vi "PreUUT Dialog.vi"(8 "error in (no error)":errorcluster, 11 "Valid Part Numbers":string[](array[string])) -> (0 "error out":errorcluster, 1 "Comments Out":string, 2 "Part Number Out":string(combo), 3 "Cancelled?":bool, 5 "Serial Number Out":string)   [LabVIEW 2020, in "Common Dialogs.lvlib"]
doc: "Use this template to create a dialog box with event handling."
uses:
  <vilib>/regexp/Match Regular Expression.xnode
  Common Dialogs.lvlib
panel:
  in  "Part Number OK":bool
  in  "Serial Number OK":bool
  in  "Comments":string
  in  "Part Number":string(combo)
  in  "Serial Number":string
  in  "Cancel":bool
  in  "OK":bool
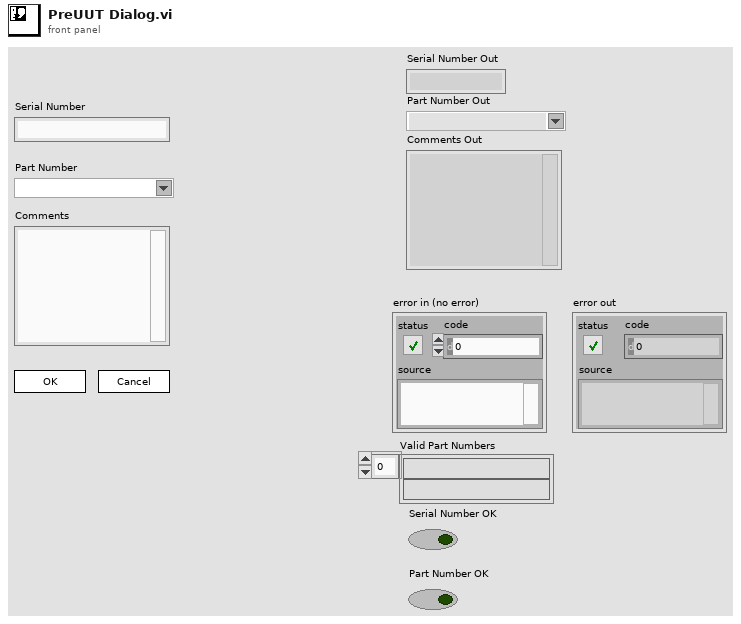
[diagram p1: front panel]
types:
  T1 = enum8{"Enabled", "Disabled", "Disabled and Grayed Out"}
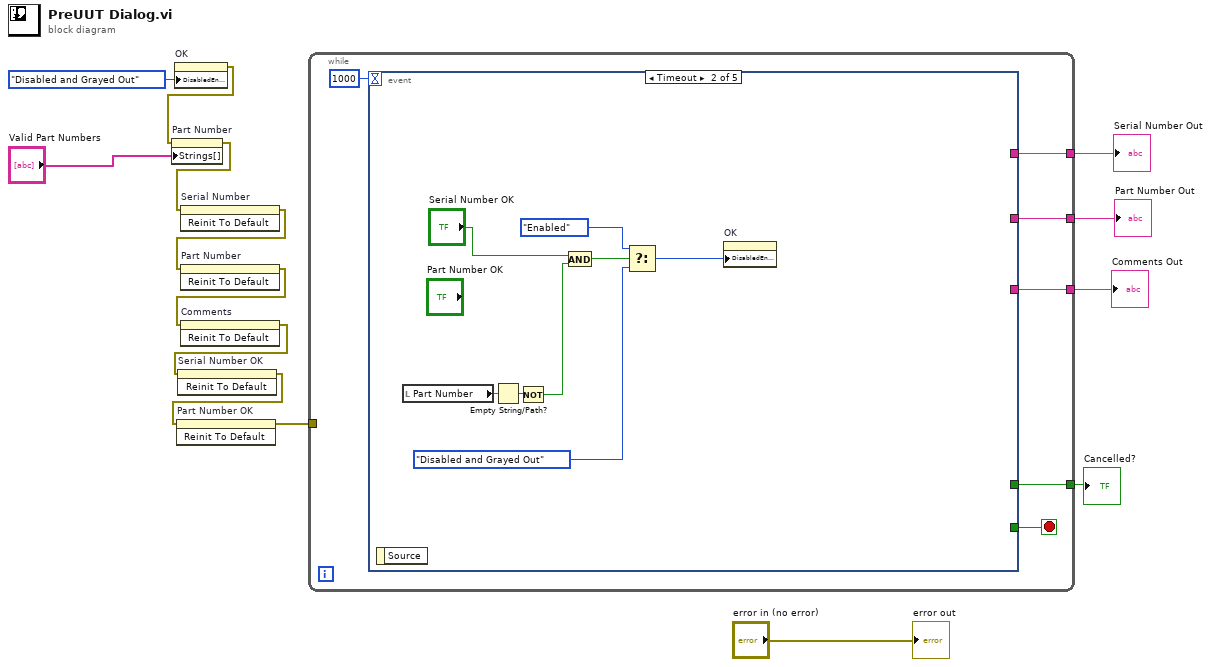
[diagram p0: block diagram]
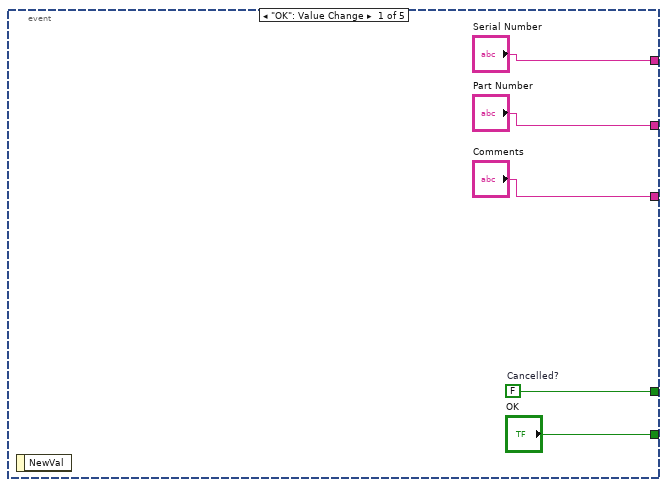
[diagram p2: hidden frame]
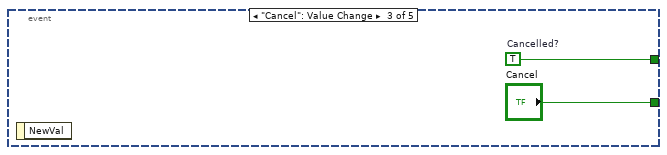
[diagram p3: hidden frame]
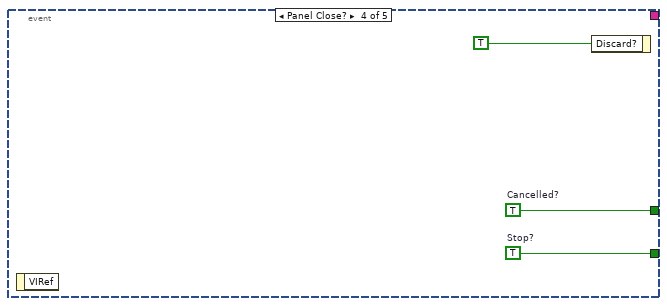
[diagram p4: hidden frame]
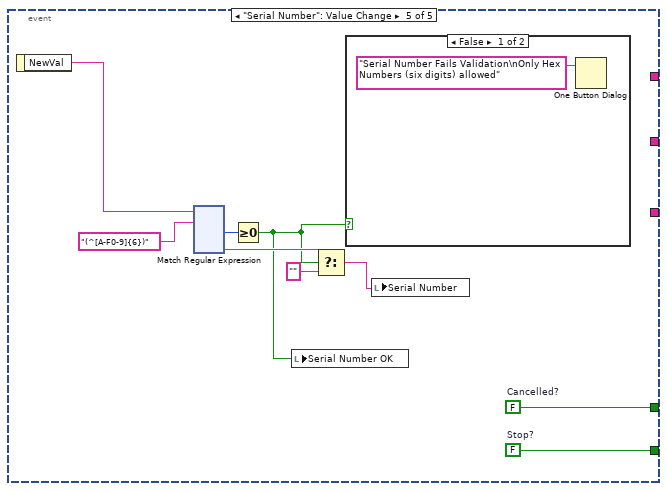
[diagram p5: hidden frame]
diagram:
  n1 = property on="OK" class="Bool"("DisabledEnum"=T1."Disabled and Grayed Out" ("Disabled")) -> (error out=w5:errorcluster)  [unwired: 2 in, 1 out]
  n2 = property on="Part Number" class="CmbBox"(error in=w5, "Strings[]"="Valid Part Numbers") -> (error out=w7:errorcluster)  [unwired: 1 in, 1 out]
  n3 = invoke on="Serial Number" class="Str" method="Reinit To Default"(error in=w7) -> (error out=w9:errorcluster)  [unwired: 2 in, 2 out]
  n4 = invoke on="Part Number" class="CmbBox" method="Reinit To Default"(error in=w9) -> (error out=w8:errorcluster)  [unwired: 2 in, 2 out]
  n5 = invoke on="Comments" class="Str" method="Reinit To Default"(error in=w8) -> (error out=w3:errorcluster)  [unwired: 2 in, 2 out]
  n6 = invoke on="Serial Number OK" class="Bool (strict)" method="Reinit To Default"(error in=w3) -> (error out=w2:errorcluster)  [unwired: 2 in, 2 out]
  n7 = invoke on="Part Number OK" class="Bool (strict)" method="Reinit To Default"(error in=w2) -> (error out=w1:errorcluster)  [unwired: 2 in, 2 out]
  n8 = while {
    tunnel: [w19] -> w14
    tunnel: [w18] -> w13
    tunnel: [w17] -> w12
    tunnel: [w16] -> w11
    tunnel: w1 -> [_]
    stop <- w20 stop-if-true
    n9 = event shown="[1] Timeout" {
      selector: _ -> [_ _ _ _ _]
      dyn-events: _ -> [_ _ _ _ _]
      timeout: 1000 -> [_ _ _ _ _]
      tunnel: ["OK" _ "Cancel" w37 w47] -> w20
      tunnel: [w25 _ w35 w36 w46] -> w19
      tunnel: ["Serial Number" _ _ _ _] -> w18
      tunnel: ["Part Number" _ _ _ _] -> w17
      tunnel: ["Comments" _ _ _ _] -> w16
      event "OK": Value Change {
        w25 = FALSE  # Cancelled?
        n10 = event-data() -> ()  [unwired: 1 in, 1 out]
      }
      event Timeout {
        n11 = event-data() -> ()  [unwired: 1 in, 1 out]
        n12 = local read "Part Number"() -> (w28:string)
        n13 = Empty String/Path?(string/path=w28) -> (empty?=w27:bool)
        n14 = Not(x=w27) -> (.not. x?=w26:bool)
        n15 = And(x="Serial Number OK", y=w26) -> (x .and. y?=w30:bool)
        n16 = Select(t=T1."Enabled" ("Disabled"), s=w30, f=T1."Disabled and Grayed Out" ("Disabled")) -> (s? t:f=w29:T1)
        n17 = property on="OK" class="Bool"("DisabledEnum"=w29) -> ()  [unwired: 2 in, 2 out]
      }
      event "Cancel": Value Change {
        w35 = TRUE  # Cancelled?
        n18 = event-data() -> ()  [unwired: 1 in, 1 out]
      }
      event Panel Close? {
        w36 = TRUE  # Cancelled?
        w37 = TRUE  # Stop?
        n19 = event-data() -> ()  [unwired: 1 in, 1 out]
        n20 = event-data("Discard?"=TRUE) -> ()  [unwired: 1 in, 1 out]
      }
      event "Serial Number": Value Change {
        w46 = FALSE  # Cancelled?
        w47 = FALSE  # Stop?
        n21 = event-data() -> ("NewVal"=w44:string)  [unwired: 1 in]
        n22 = xnode "Match Regular Expression"("input string"=w44, "regular expression"="(^[A-F0-9]{6})") -> ("offset past match"=w45:i32, "submatch 1"=w42:string)  [unwired: 4 in, 4 out]
        n23 = Greater Or Equal To 0?(x=w45) -> (x >= 0?=w39:bool)
        n24 = local write "Serial Number OK"(w39) -> ()
        n25 = Select(t=w42, s=w39, f="") -> (s? t:f=w40:string)
        n26 = case shown="False" w39 {
          frame False {
            n27 = One Button Dialog(message="Serial Number Fails Validation\nOnly Hex Numbers (six digits) allowed") -> ()  [unwired: 1 in, 1 out]
          }
          frame True {
          }
        }
        n28 = local write "Serial Number"(w40) -> ()
      }
    }
  }
  "Cancelled?" <- w14
  "Serial Number Out" <- w13
  "Part Number Out" <- w12
  "Comments Out" <- w11
  "error out" <- "error in (no error)"
